vi "Marvin.vi"() -> ()   [LabVIEW 2017]
uses:
  PCAN_Driver/ControlCAN.llb/CAN Channel.ctl
  PCAN_Driver/ControlCAN.llb/DevType.ctl
  PCAN_Driver/ControlCAN.llb/VCI_INIT_CONFIG.ctl
  PCAN_Driver/ControlCAN.llb/InitFlag.ctl
  PCAN_Driver/ControlCAN.llb/Fliter.ctl
  PCAN_Driver/ControlCAN.llb/Mode.ctl
  <vilib>/Utility/miscctls.llb/LVMinMaxIncTypeDef.ctl
  PCAN_Driver/ControlCAN.llb/VCI_CAN_OBJ.ctl
  PCAN_Driver/ControlCAN.lvlib
panel:
  out "Array":u64[][](array[numeric]) format="%016x"
  out "Waveform Chart":dbl[](graph)
  out "Ambient Over temp":bool
  out "Ambient Sensor temp":bool
  out "Ambient Temperature":dbl
  in  "Motor Over Temp":bool
  in  "Speed control":bool
  out "Unit Adress":string
  in  "Serial Send":bool
  in  "Index":u16(ring) items=["1"=1, "2"=2, "3"=3]
  out "read buffer":string
  in  "SetGet":enum16{"Get", "Set"}(ring)
  in  "Function":T1(ring)
  in  "Value":dbl
  in  "Value 1/2":enum16{"1", "2"}(ring)
  out "Msg Count":u32
  in  "Param to Set":u16(ring) items=["EBAY 5F"=95, "AHU 3F"=63, "AHU 2F"=47]
  out "Unit Adress":u8
  out "Horizontal Progress Bar":i32(slide) min=0 max=48 scale=0.0..50.0
  out "character string":string
  in  "Set Param.":bool
  in  "Serial Monitor":bool caption="Graph Button"
  in  "Serial Com":bool
  in  "VISA resource name":refnum<visa-resource-name>="COM6"
  out "Serial Status":bool
  in  "Graph Button":bool
  in  "Refresh Button":bool
  out "Data Send":u64 format="%016x"
  in  "Motor Speed RPM":u16
  out "Under voltage/Over voltage":bool
  out "Speed error":bool
  out "Derated drive temp":bool
  out "Motor Over temperature":bool
  out "Commutation err":bool
  out "Motor Sensor temp Fauilre":bool
  out "Drive Over temperature":bool
  out "Drive Sensor temp Failure":bool
  out "Motor Phase Current RMS":dbl
  out "ECS State":u16
  out "Motor Speed RPM":dbl
  out "Motor Stator Temp.":dbl
  out "Power transistor Heat sink Temp.":dbl
  out "DC Current":dbl
  out "DC Voltage":dbl
  in  "Can Send":bool
  in  "Stop":bool
  out "Config_CANAT":T8 {"DevType" items=["USB-CAN"=3, "USB-CAN2"=4]; "CanIndex" items=["通道1", "通道2"]; "VCI_INIT_CONFIG"."Fliter" items=["接收所有类型"=3, "只接收标准帧"=4, "只接收扩展帧"=7]; "VCI_INIT_CONFIG"."Mode" items=["正常工作", "自测模式（环回）", "仅侦听模式"]; "VCI_INIT_CONFIG"."InitFlag" items=["使用Flash参数", "使用界面设置参数"]}
  in  "Channel 2":T3 caption="Channel" items=["Channel 1", "Channel 2"]
  out "CAN Status":bool
  # "ver 1.0"
  # "Marvin"
  # "REDLER TECHNOLOGIES LTD"
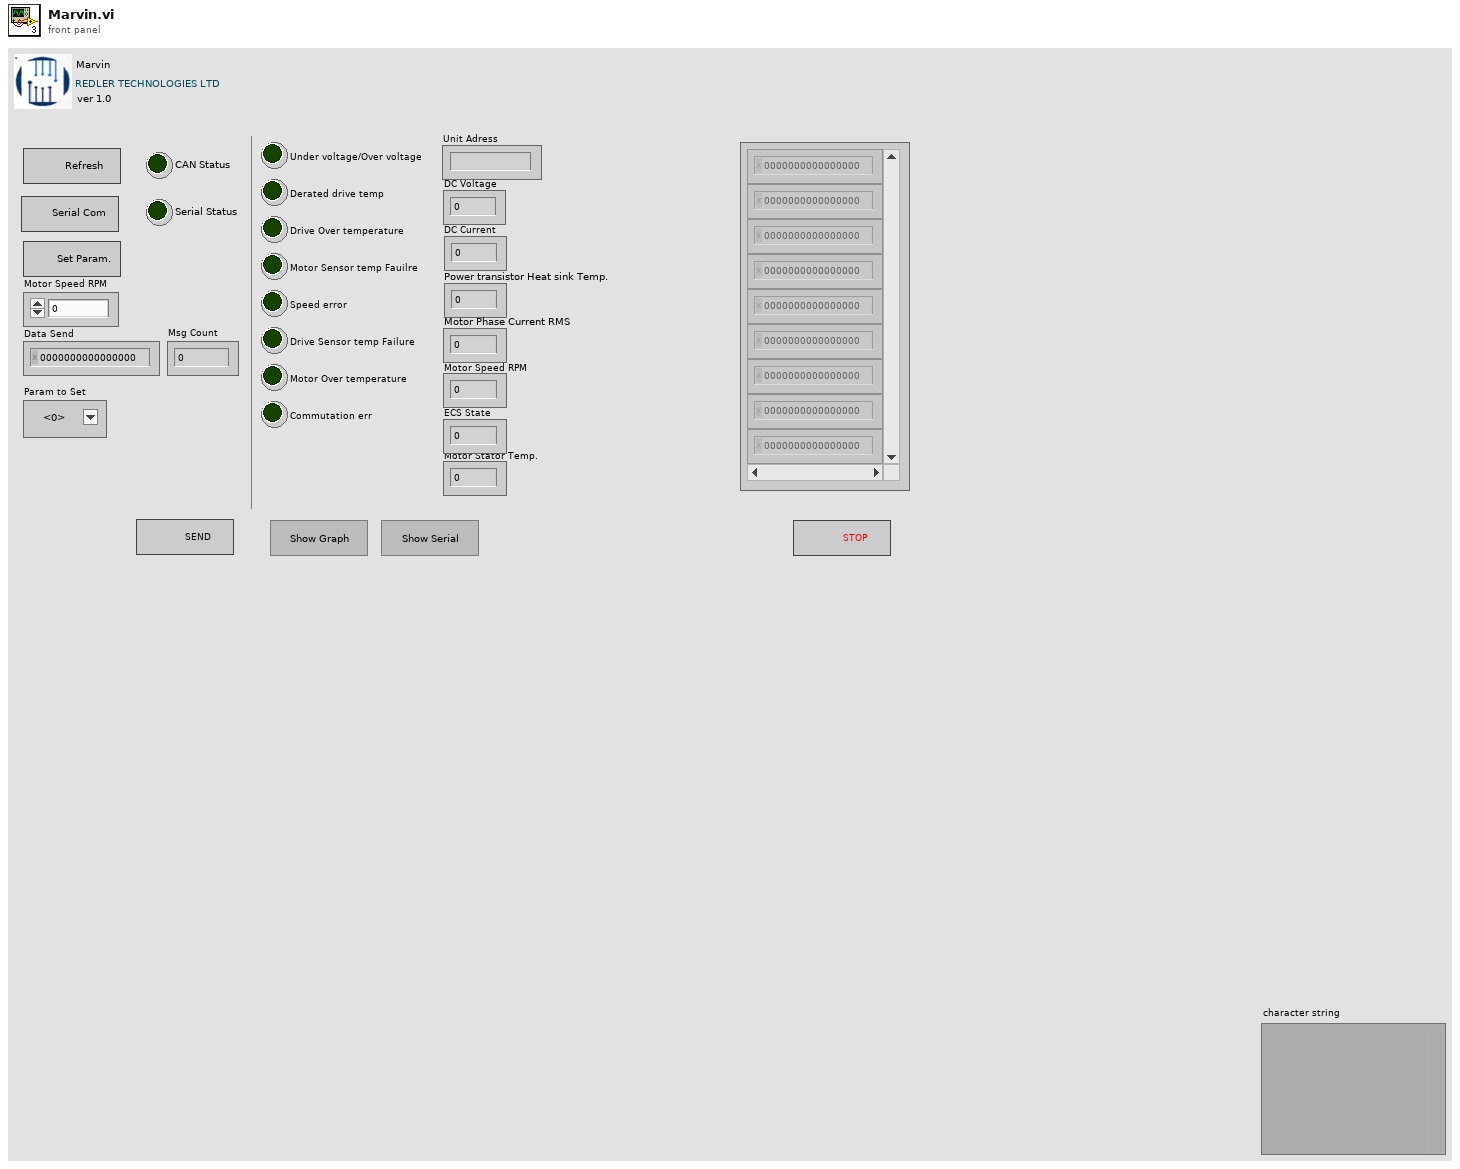
[diagram p1: front panel]
types:
  T1 = enum16{"Serial Number", "Temperature", "Unit Adress", "Calibration", "Velocity", "Version"}
  T2 = typedef "ControlCAN.lvlib/DevType.ctl" = u32
  T3 = typedef "ControlCAN.lvlib/CAN Channel.ctl" = u32
  T4 = typedef "ControlCAN.lvlib/VCI_INIT_CONFIG.ctl" = cluster{"AccCode":u32, "AccMask":u32, "InitFlag":T5, "Fliter":T6, "Timing0":u8, "Timing1":u8, "Mode":T7}
  T5 = typedef "ControlCAN.lvlib/InitFlag.ctl" = u32
  T6 = typedef "ControlCAN.lvlib/Fliter.ctl" = u8
  T7 = typedef "ControlCAN.lvlib/Mode.ctl" = u8
  T8 = cluster{"DevType":T2, "DevIndex":u32, "CanIndex":T3, "VCI_INIT_CONFIG":T4}
  T9 = cluster{"ID":u32, "MSGTYPE":u8, "LEN":u8, "aDATA":u8[]}[]
  T10 = cluster{"ID":u32, "MSGTYPE":u8, "LEN":u8, "aDATA":u8[]}
  T11 = enum8{"Enabled", "Disabled", "Disabled and Grayed Out"}
  T12 = typedef "LVMinMaxIncTypeDef.ctl" = cluster{"Minimum":dbl, "Maximum":dbl, "Increment":dbl}
  T13 = typedef "ControlCAN.lvlib/VCI_CAN_OBJ.ctl" = cluster{"ID":u32, "TimeStamp":u32, "TimeFlag":u8, "SendType":u8, "RemoteFlag":u8, "ExternFlag":u8, "DataLen":u8, "Data":u8[], "Reserved":u8[]}
  T14 = cluster{"Type":enum16{"接收", "发送"}, "Channel":T3, "Time":timestamp, "VCI_CAN_OBJ":T13}[]
  T15 = cluster{"Type":enum16{"接收", "发送"}, "Channel":T3, "Time":timestamp, "VCI_CAN_OBJ":T13}
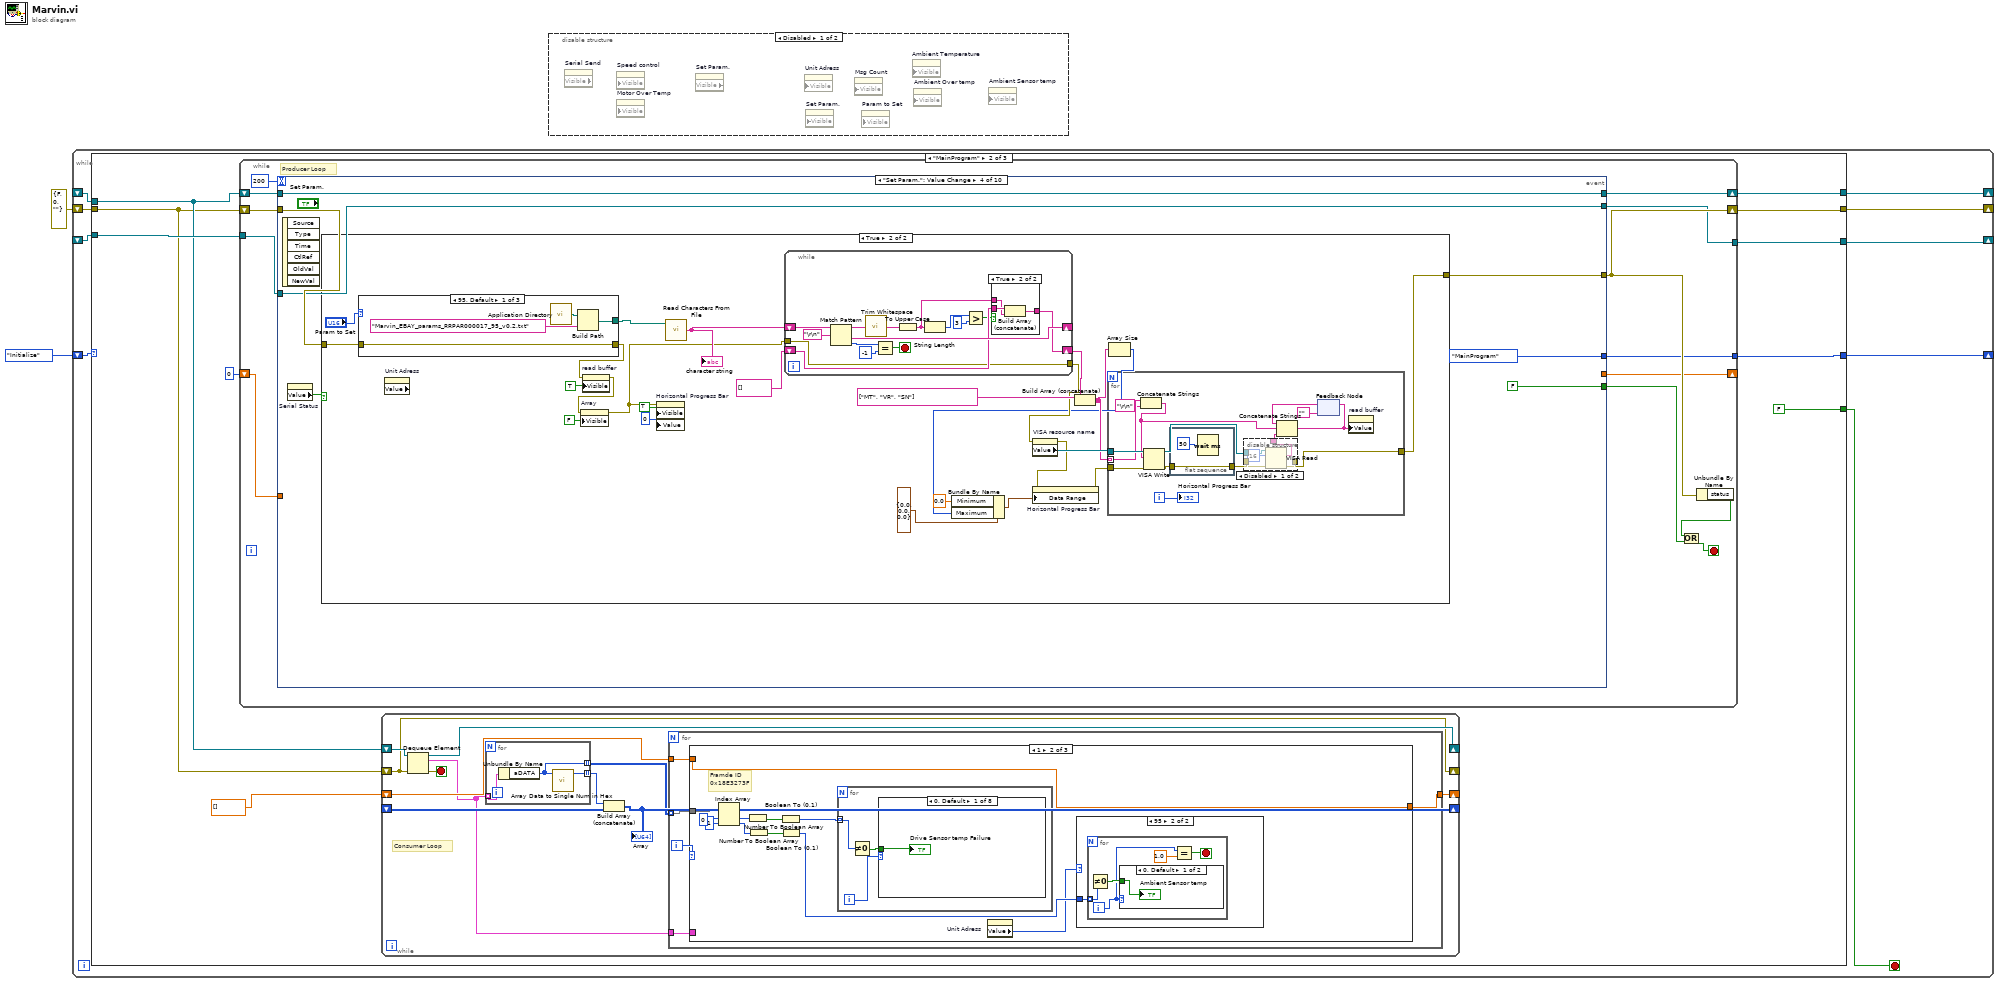
[diagram p0: block diagram]
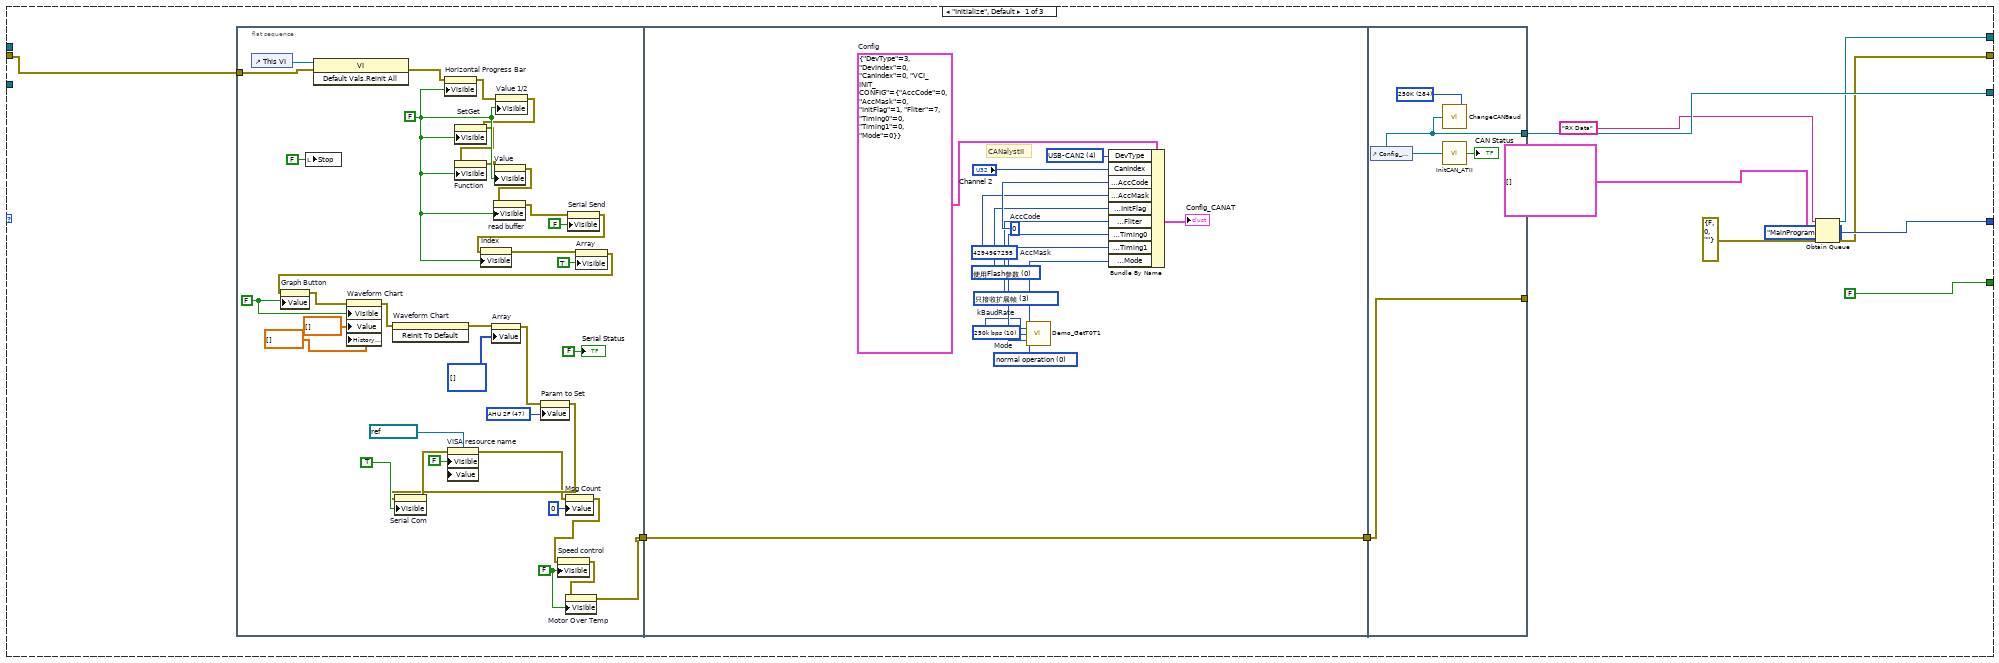
[diagram p3: hidden frame]
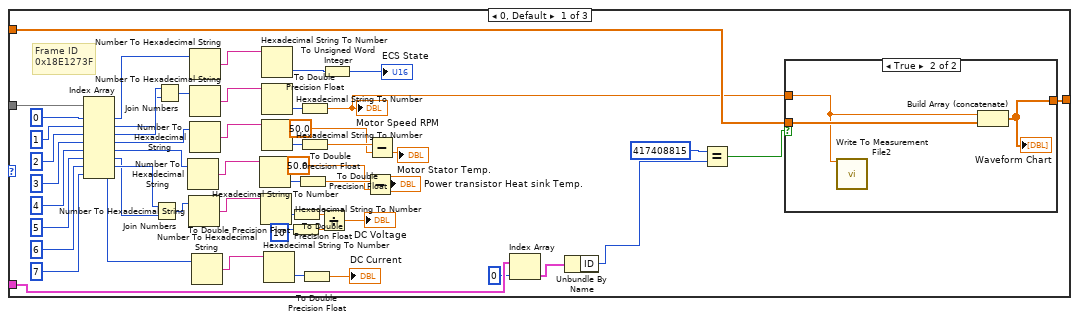
[diagram p4: hidden frame]
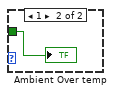
[diagram p7: hidden frame]
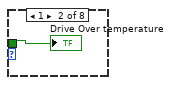
[diagram p8: hidden frame]
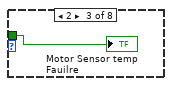
[diagram p9: hidden frame]
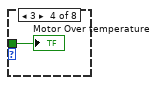
[diagram p10: hidden frame]
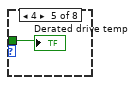
[diagram p11: hidden frame]
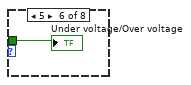
[diagram p12: hidden frame]
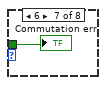
[diagram p13: hidden frame]
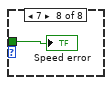
[diagram p14: hidden frame]
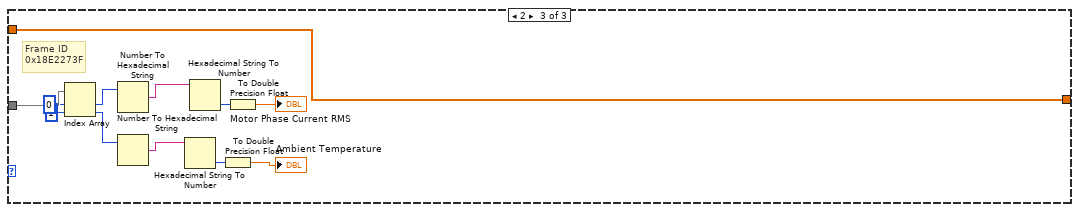
[diagram p15: hidden frame]
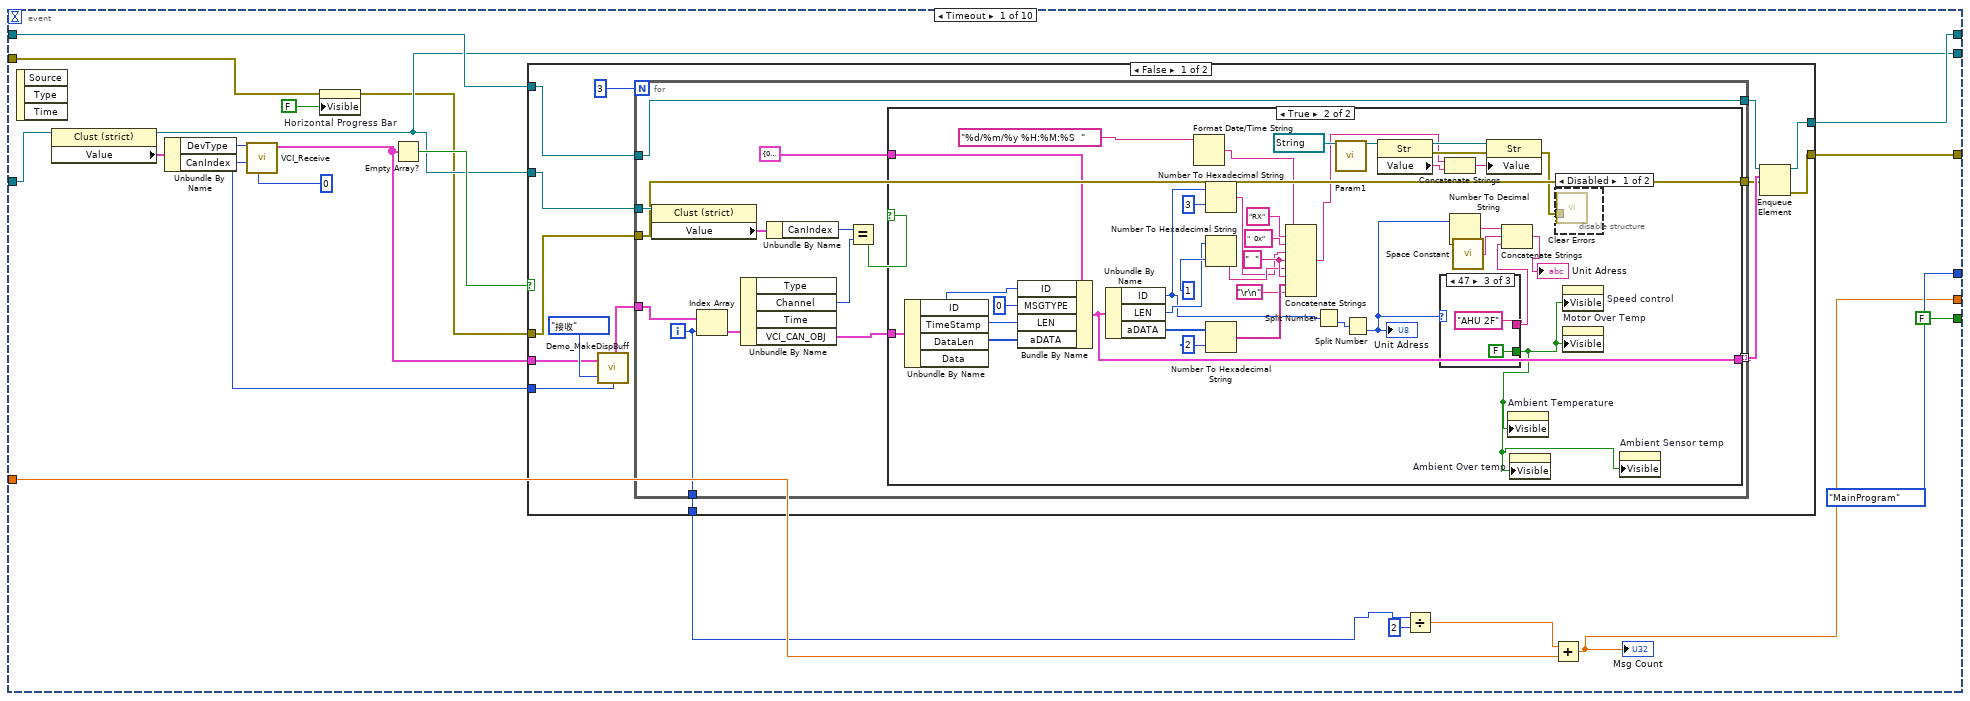
[diagram p16: hidden frame]
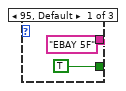
[diagram p18: hidden frame]
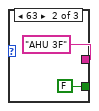
[diagram p19: hidden frame]
diagram:
  n1 = while {
    shift-right: [w6] -> _
    shift-left: enum16{"Stop", "MainProgram", "Initialize"}."Initialize" -> [w11]
    shift-right: [w10] -> _
    shift-left: _ -> [w9]
    shift-right: [w8] -> _
    shift-left: _ -> [w5]
    shift-right: [w7] -> _
    shift-left: errorcluster {"status"=FALSE, "code"=0, "source"=""} ("error out") -> [w4]
    stop <- w3 stop-if-true
    n2 = case shown="\"MainProgram\"" w11 {
      tunnel: [w22 w83 w734] -> w10
      tunnel: w9 -> [_ w86 w734]
      tunnel: [w18 w85 w735] -> w8
      tunnel: [w17 w84 w736] -> w7
      tunnel: [enum16{"Stop", "MainProgram", "Initialize"}."MainProgram" w82 enum16{"Stop", "MainProgram", "Initialize"}."Stop"] -> w6
      tunnel: w5 -> [_ w81 w735]
      tunnel: w4 -> [w15 w80 w737]
      tunnel: [FALSE ("Stop") FALSE ("Stop") w733] -> w3
      frame "Initialize", Default {
        n3 = flat-sequence {
          tunnel: w15 -> [w28]
          tunnel: [w24] -> w13
          tunnel: [w60] -> w14
          tunnel: w13 -> [w60]
          tunnel: [w74] -> w22
          tunnel: w14 -> [w73]
          tunnel: [w73] -> _
          frame #0 {
            w23 = FALSE ("Visible")
            w43 = u16 47 items=["EBAY 5F"=95, "AHU 3F"=63, "AHU 2F"=47] ("Param to Set")
            w46 = FALSE ("Visible")
            w50 = FALSE ("Graph Button")
            n4 = control-ref of="This VI"() -> (w59:refnum<vi>)
            n5 = local write "Stop"(FALSE ("Stop")) -> ()
            n6 = invoke class="VI" method="Default Vals.Reinit All"(reference=w59, error in=w28) -> (error out=w27:errorcluster)  [unwired: 1 in, 2 out]
            n7 = property on="Horizontal Progress Bar" class="Slide (strict)"(error in=w27, "Visible"=w46) -> (error out=w41:errorcluster)  [unwired: 1 in, 1 out]
            n8 = property on="Value 1/2" class="Enum (strict)"(error in=w41, "Visible"=w46) -> (error out=w40:errorcluster)  [unwired: 1 in, 1 out]
            n9 = property on="SetGet" class="Enum (strict)"(error in=w40, "Visible"=w46) -> (error out=w39:errorcluster)  [unwired: 1 in, 1 out]
            n10 = property on="Function" class="Enum (strict)"(error in=w39, "Visible"=w46) -> (error out=w38:errorcluster)  [unwired: 1 in, 1 out]
            n11 = property on="Value" class="DigNum (strict)"(error in=w38, "Visible"=w46) -> (error out=w37:errorcluster)  [unwired: 1 in, 1 out]
            n12 = property on="read buffer" class="Str"(error in=w37, "Visible"=w46) -> (error out=w36:errorcluster)  [unwired: 1 in, 1 out]
            n13 = property on="Serial Send" class="Bool"(error in=w36, "Visible"=FALSE) -> (error out=w35:errorcluster)  [unwired: 1 in, 1 out]
            n14 = property on="Index" class="Ring (strict)"(error in=w35, "Visible"=w46) -> (error out=w34:errorcluster)  [unwired: 1 in, 1 out]
            n15 = property on="Array" class="Arr (strict)"(error in=w34, "Visible"=TRUE) -> (error out=w33:errorcluster)  [unwired: 1 in, 1 out]
            n16 = property on="Graph Button" class="Bool (strict)"(error in=w33, "Value"=w50) -> (error out=w32:errorcluster)  [unwired: 1 in, 1 out]
            n17 = property on="Waveform Chart" class="WFChart (strict)"(error in=w32, "Visible"=w50, "Value"=dbl[] [] ("Waveform Chart"), "History Data"=dbl[] []) -> (error out=w53:errorcluster)  [unwired: 1 in, 1 out]
            n18 = invoke on="Waveform Chart" class="WFChart (strict)" method="Reinit To Default"(error in=w53) -> (error out=w54:errorcluster)  [unwired: 2 in, 2 out]
            n19 = property on="Array" class="Arr (strict)"(error in=w54, "Value"=u64[][] [] ("Array")) -> (error out=w31:errorcluster)  [unwired: 1 in, 1 out]
            n20 = property on="Param to Set" class="Ring (strict)"(error in=w31, "Value"=w43) -> (error out=w30:errorcluster)  [unwired: 1 in, 1 out]
            n21 = property on="Serial Com" class="Bool"(error in=w30, "Visible"=TRUE) -> (error out=w56:errorcluster)  [unwired: 1 in, 1 out]
            n22 = property on="VISA resource name" class="VISAName"(error in=w56, "Visible"=FALSE, "Value"=refnum<visa-resource-name> "COM1" ("VISA resource name")) -> (error out=w29:errorcluster)  [unwired: 1 in, 1 out]
            n23 = property on="Msg Count" class="DigNum (strict)"(error in=w29, "Value"=u32 0 ("Msg Count")) -> (error out=w26:errorcluster)  [unwired: 1 in, 1 out]
            n24 = property on="Speed control" class="Bool (strict)"(error in=w26, "Visible"=w23) -> (error out=w25:errorcluster)  [unwired: 1 in, 1 out]
            n25 = property on="Motor Over Temp" class="Bool (strict)"(error in=w25, "Visible"=w23) -> (error out=w24:errorcluster)  [unwired: 1 in, 1 out]
            "Serial Status" <- FALSE ("Serial Status")
          }
          frame #1 {
            w64 = u32 4294967295  # AccMask
            w63 = T5 0 items=["使用Flash参数", "使用界面设置参数"] ("InitFlag")
            w61 = T7 0 items=["normal operation", "Listen-only mode", "test mode"]  # Mode
            w62 = T6 3 items=["接收所有类型"=1, "只接收标准帧"=2, "只接收扩展帧"=3] ("Fliter")
            w68 = u8 10 items=["5k bps"=1, "10k bps"=2, "20k bps"=3, "40k bps"=4, "50k bps"=5, "80k bps"=6, "100k bps"=7, "125k bps"=8, "200k bps"=9, "250k bps"=10, "400k bps"=11, "500k bps"=12, "666k bps"=13, "800k bps"=14, "1000k bps"=15, "33.33k bps"=16, "66.66k bps"=17, "83.33k bps"=18]  # kBaudRate
            w65 = u32 0  # AccCode
            w66 = T2 4 items=["USB-CAN"=3, "USB-CAN2"=4] ("DevType")
            w67 = T8 {"DevType"=3, "DevIndex"=0, "CanIndex"=0, "VCI_INIT_CONFIG"={"AccCode"=0, "AccMask"=0, "InitFlag"=1, "Fliter"=7, "Timing0"=0, "Timing1"=0, "Mode"=0}}  # Config
            # "CANalystII"
            n26 = call "Demo_GetT0T1.vi"("kBaudRate"=w68) -> ("Timing0"=w70:u8, "Timing1"=w71:u8)
            n27 = Bundle By Name(cluster=w67, "DevType"=w66, "CanIndex"="Channel 2", "VCI_INIT_CONFIG.AccCode"=w65, "VCI_INIT_CONFIG.AccMask"=w64, "VCI_INIT_CONFIG.InitFlag"=w63, "VCI_INIT_CONFIG.Fliter"=w62, "VCI_INIT_CONFIG.Timing0"=w70, "VCI_INIT_CONFIG.Timing1"=w71, "VCI_INIT_CONFIG.Mode"=w61) -> (→"Config_CANAT":T8)
          }
          frame #2 {
            w75 = u16 284 items=["1M"=20, "500K"=28, "250K"=284, "125K"=796, "100K"=17199, "50K"=18223, "20K"=21295, "10K"=26415, "5K"=32639] ("baud in")
            n28 = control-ref of="Config_CANAT"() -> (w74:refnum<vi>)
            n29 = call "ChangeCANBaud.vi"("baud in"=w75, "reference"=w74) -> ()
            n30 = call "InitCAN_ATII.vi"("Config"=w74) -> ("Sts"=→"CAN Status":bool)
          }
        }
        n31 = Obtain Queue(name (unnamed)="RX Data", element data type=T9 [], error in (no error)=errorcluster {"status"=FALSE, "code"=0, "source"=""}) -> (queue out=w18:refnum<queue>, error out=w17:errorcluster)  [unwired: 2 in, 1 out]
      }
      frame "MainProgram" {
        n32 = while {
          shift-right: [w210] -> w84
          shift-left: w80 -> [w212]
          shift-right: [w211] -> w85
          shift-left: w81 -> [w213]
          tunnel: w86 -> [w214]
          tunnel: [w207] -> w83
          tunnel: [w206] -> w82
          shift-right: [w204] -> _
          shift-left: 0 -> [w205]
          stop <- w215 stop-if-true
          # "Producer Loop"
          n33 = event shown="[3] \"Set Param.\": Value Change" {
            selector: _ -> [_ _ _ _ _ _ _ _ _ _]
            dyn-events: _ -> [_ _ _ _ _ _ _ _ _ _]
            timeout: 200 -> [_ _ _ _ _ _ _ _ _ _]
            tunnel: w214 -> [w234 w315 w356 w542 w636 w686 w698 w711 w725 w730]
            tunnel: w213 -> [w231 w319 w357 w541 w657 w687 w697 w712 w722 w727]
            tunnel: w212 -> [w223 w316 w358 w543 w656 w688 w693 w704 w721 w728]
            tunnel: [w229 w319 w357 w541 w657 w687 w697 w712 w720 w727] -> w211
            tunnel: [w228 w314 w355 w538 w656 w688 w690 w701 w718 w726] -> w210
            tunnel: [FALSE ("Stop") FALSE ("Stop") FALSE ("Stop") FALSE ("Stop") FALSE ("Stop") FALSE ("Stop") FALSE ("Stop") FALSE ("Stop") TRUE ("Stop") TRUE ("Stop")] -> w208
            tunnel: [w227 w315 w356 w542 w636 w686 w698 w711 w725 w730] -> w207
            tunnel: [enum16{"Stop", "MainProgram", "Initialize"}."MainProgram" enum16{"Stop", "MainProgram", "Initialize"}."MainProgram" enum16{"Stop", "MainProgram", "Initialize"}."MainProgram" enum16{"Stop", "MainProgram", "Initialize"}."MainProgram" enum16{"Stop", "MainProgram", "Initialize"}."MainProgram" enum16{"Stop", "MainProgram", "Initialize"}."MainProgram" enum16{"Stop", "MainProgram", "Initialize"}."MainProgram" enum16{"Stop", "MainProgram", "Initialize"}."MainProgram" enum16{"Stop", "MainProgram", "Initialize"}."Stop" enum16{"Stop", "MainProgram", "Initialize"}."Initialize"] -> w206
            tunnel: w205 -> [w222 _ _ _ _ _ _ _ _ _]
            tunnel: [w221 _ _ _ _ _ _ _ _ _] -> w204
            event Timeout {
              n34 = event-data() -> ()  [unwired: 1 in, 3 out]
              n35 = property class="Clust (strict)"(reference=w234) -> (reference out=w227:refnum<vi>, "Value"=w235:T8)  [unwired: 1 in, 1 out]
              n36 = Unbundle By Name(w235) -> ("DevType"=w236:T2, "CanIndex"=w232:T3)
              n37 = call "VCI_Receive.vi"("CANIndex"=w232, "DevIndex"=u32 0, "DevType"=w236) -> ("Recieve"=w230:T13[])  [unwired: 3 in, 5 out]
              n38 = property on="Horizontal Progress Bar" class="Slide (strict)"(error in=w223, "Visible"=FALSE) -> (error out=w217:errorcluster)  [unwired: 1 in, 1 out]
              n39 = Empty Array?(array=w230) -> (empty?=w233:bool)
              n40 = case shown="False" w233 {
                tunnel: w232 -> [w249 _]
                tunnel: w227 -> [w247 _]
                tunnel: w231 -> [w246 w312]
                tunnel: w217 -> [w245 w311]
                tunnel: w230 -> [w250 _]
                tunnel: [w240 w311] -> w228
                tunnel: [w239 w312] -> w229
                tunnel: [w238 0] -> w218
                frame False {
                  n41 = call "Demo_MakeDispBuff.vi"("Channel"=w249, "Type"=enum16{"接收", "发送"}."接收", "OBJs"=w250) -> ("Buffer"=w248:T14)
                  n42 = for {
                    N: 3 -> [_]
                    tunnel: w248 -> [w264]
                    tunnel: w247 -> [w263]
                    tunnel: w246 -> [w254]
                    tunnel: w245 -> [w253]
                    tunnel: [w256] -> w243 mode=indexing
                    tunnel: [w254] -> w242
                    tunnel: [w253] -> w241
                    tunnel: [w252] -> w238
                    i -> [w252]
                    n43 = property class="Clust (strict)"(reference=w263) -> ("Value"=w261:T8)  [unwired: 1 in, 2 out]
                    n44 = Index Array(array=w264, index=w252) -> (element=w257:T15)
                    n45 = Unbundle By Name(w257) -> ("Channel"=w259:T3, "VCI_CAN_OBJ"=w262:T13)  [unwired: 2 out]
                    n46 = Unbundle By Name(w261) -> ("CanIndex"=w260:T3)
                    n47 = Equal?(x=w260, y=w259) -> (x = y?=w258:bool)
                    n48 = case shown="True" w258 {
                      tunnel: w262 -> [_ w302]
                      tunnel: [w265 w278] -> w256
                      tunnel: T10 {"ID"=0, "MSGTYPE"=0, "LEN"=0, "aDATA"=[]} ("Msg") -> [w265 w277]
                      frame False {
                      }
                      frame True {
                        w289 = "  " ("string")
                        n49 = Unbundle By Name(w302) -> ("ID"=w274:u32, "DataLen"=w301:u8, "Data"=w279:u8[])  [unwired: 1 out]
                        n50 = Bundle By Name(cluster=w277, "ID"=w274, "MSGTYPE"=u8 0, "LEN"=w301, "aDATA"=w279) -> (w278:T10)
                        n51 = Unbundle By Name(w278) -> ("ID"=w272:u32, "LEN"=w284:u8, "aDATA"=w290:u8[])
                        n52 = Format Date/Time String(time format string (%c)="%d/%m/%y %H:%M:%S  ") -> (date/time string=w299:string)  [unwired: 2 in]
                        n53 = Number To Hexadecimal String(1:i16 3 ("width (-)"), 2:w272) -> (0:w276:string)
                        n54 = Number To Hexadecimal String(1:i16 1 ("width (-)"), 2:w284) -> (0:w288:string)
                        n55 = Number To Hexadecimal String(1:i16 2 ("width (-)"), 2:w290) -> (0:w291:string[])
                        n56 = Concatenate Strings(w299, "RX" ("string"), "  0x" ("string"), w276, w289, w288, w289, w291, "\r\n") -> (w275:string)
                        n57 = Split Number(x=w272) -> (lo(x)=w273:u16)  [unwired: 1 out]
                        n58 = call "Param1.vi"("str"=refnum<vi> refnum) -> ("str out"=w293:refnum<vi>)  [unwired: 17 in, 1 out]
                        n59 = Split Number(x=w273) -> (lo(x)=w271:u8)  [unwired: 1 out]
                        "Unit Adress" <- w271
                        n60 = property class="Str"(reference=w293) -> (reference out=w295:refnum<vi>, error out=w281:errorcluster, "Value"=w296:string)  [unwired: 1 in]
                        n61 = case shown="47" w271 {
                          tunnel: ["EBAY 5F" "AHU 3F" "AHU 2F"] -> w269
                          tunnel: [TRUE FALSE FALSE] -> w266
                          frame 95, Default {
                          }
                          frame 63 {
                          }
                          frame 47 {
                          }
                        }
                        n62 = Concatenate Strings(w275, w296) -> (w294:string)
                        n63 = Number To Decimal String(number=w271) -> (decimal integer string=w270:string)  [unwired: 1 in]
                        n64 = call <vilib>:"Space Constant.vi"() -> ("String"=w267:string)
                        n65 = property class="Str"(reference=w295, error in=w281, "Value"=w294) -> (error out=w280:errorcluster)  [unwired: 1 out]
                        n66 = Concatenate Strings(w270, w267, w269) -> (→"Unit Adress":string)
                        n67 = property on="Ambient Temperature" class="DigNum (strict)"("Visible"=w266) -> ()  [unwired: 2 in, 2 out]
                        n68 = property on="Ambient Over temp" class="Bool (strict)"("Visible"=w266) -> ()  [unwired: 2 in, 2 out]
                        n69 = disable-structure shown="Disabled" {
                          disable-tunnel: w280 -> [w309 _]
                          frame Disabled {
                            n70 = call <vilib>:"Clear Errors.vi"("error in (no error)"=w309) -> ()  [unwired: 5 in, 2 out]
                          }
                          frame Enabled {
                          }
                        }
                        n71 = property on="Speed control" class="Bool (strict)"("Visible"=w266) -> ()  [unwired: 2 in, 2 out]
                        n72 = property on="Motor Over Temp" class="Bool (strict)"("Visible"=w266) -> ()  [unwired: 2 in, 2 out]
                        n73 = property on="Ambient Sensor temp" class="Bool (strict)"("Visible"=w266) -> ()  [unwired: 2 in, 2 out]
                      }
                    }
                  }
                  n74 = Enqueue Element(queue=w242, element=w243, error in (no error)=w241) -> (queue out=w239:refnum<queue>, error out=w240:errorcluster)  [unwired: 2 out]
                }
                frame True {
                }
              }
              n75 = Divide(x=w218, y=u32 2) -> (x/y=w219:dbl)
              n76 = Add(x=w219, y=w222) -> (x+y=w221:dbl)
              "Msg Count" <- w221
            }
            event "Serial Monitor": Value Change {
              n77 = event-data() -> ()  [unwired: 1 in, 6 out]
              n78 = property on="Serial Status" class="Bool (strict)"() -> ("Value"=w313:bool)  [unwired: 2 in, 2 out]
              n79 = case shown="True" w313 {
                tunnel: w316 -> [w321 w332]
                tunnel: [w320 w338] -> w314
                frame False {
                  n80 = call "Display Message to User3"("error in (no error)"=w321) -> ("error out"=w320:errorcluster)  [unwired: 9 in, 1 out]
                }
                frame True {
                  w334 = FALSE ("Visible")
                  w335 = u16 1 items=["1"=1, "2"=2, "3"=3] ("Index")
                  n81 = property on="Index" class="Ring (strict)"(error in=w332, "Value"=w335) -> (error out=w331:errorcluster)  [unwired: 1 in, 1 out]
                  n82 = property on="Value 1/2" class="Enum (strict)"(error in=w331, "Visible"=w334) -> (error out=w330:errorcluster)  [unwired: 1 in, 1 out]
                  n83 = property on="Value" class="DigNum (strict)"(error in=w330, "Visible"=w334) -> (error out=w329:errorcluster)  [unwired: 1 in, 1 out]
                  n84 = property on="SetGet" class="Enum (strict)"(error in=w329, "Value"=enum16{"Get", "Set"}."Get" ("SetGet")) -> (error out=w327:errorcluster)  [unwired: 1 in, 1 out]
                  n85 = property on="Serial Send" class="Bool"(error in=w327, "Visible"=FALSE) -> (error out=w326:errorcluster)  [unwired: 1 in, 1 out]
                  n86 = property on="Function" class="Enum (strict)"(error in=w326, "Value"=T1."Serial Number" ("Function")) -> (error out=w324:errorcluster)  [unwired: 1 in, 1 out]
                  n87 = property on="Index" class="Ring (strict)"(error in=w324, "DisabledEnum"=T11."Disabled and Grayed Out" ("Disabled")) -> (error out=w322:errorcluster)  [unwired: 1 in, 1 out]
                  n88 = case shown="False" "Serial Monitor" {
                    selector: "Serial Monitor" -> [w339 w345]
                    tunnel: w322 -> [w343 w350]
                    tunnel: [w342 w348] -> w338
                    tunnel: [FALSE TRUE] -> w336
                    frame False {
                      (unwired) FALSE ("Visible")
                      n89 = Not(x=w339) -> (.not. x?=w340:bool)
                      n90 = property on="Array" class="Arr (strict)"(error in=w343, "Visible"=w340) -> (error out=w344:errorcluster)  [unwired: 1 in, 1 out]
                      n91 = property on="Serial Monitor" class="Bool (strict)"(error in=w344, "Value"=w339) -> (error out=w342:errorcluster)  [unwired: 1 in, 1 out]
                    }
                    frame True {
                      (unwired) FALSE ("Visible")
                      n92 = Not(x=w345) -> (.not. x?=w346:bool)
                      n93 = property on="Array" class="Arr (strict)"(error in=w350, "Visible"=w346) -> (error out=w349:errorcluster)  [unwired: 1 in, 1 out]
                      n94 = property on="Serial Monitor" class="Bool (strict)"(error in=w349, "Value"=w345) -> (error out=w348:errorcluster)  [unwired: 1 in, 1 out]
                    }
                  }
                  n95 = property on="SetGet" class="Enum (strict)"("Visible"=w336) -> ()  [unwired: 2 in, 2 out]
                  n96 = property on="Function" class="Enum (strict)"("Visible"=w336) -> ()  [unwired: 2 in, 2 out]
                  n97 = property on="Serial Send" class="Bool"("Visible"=w336) -> ()  [unwired: 2 in, 2 out]
                  n98 = property on="read buffer" class="Str"("Visible"=w336) -> ()  [unwired: 2 in, 2 out]
                  n99 = property on="Index" class="Ring (strict)"("Visible"=w336) -> ()  [unwired: 2 in, 2 out]
                }
              }
            }
            event "Serial Send": Value Change {
              n100 = event-data() -> ()  [unwired: 1 in, 6 out]
              n101 = property on="VISA resource name" class="VISAName"() -> ("Value"=w359:refnum<visa-resource-name>)  [unwired: 2 in, 2 out]
              n102 = case shown="\"Set\"" "SetGet" {
                tunnel: "Function" -> [w365 w444]
                tunnel: w359 -> [w373 w459]
                tunnel: w358 -> [w369 w443]
                tunnel: "Value" -> [_ w458]
                tunnel: "Value 1/2" -> [_ w456]
                tunnel: "Index" -> [w366 w453]
                tunnel: [w372 w451] -> _
                tunnel: [w371 w450] -> w355
                tunnel: [w367 w448] -> w354
                frame "Get", Default {
                  w370 = FALSE ("Visible")
                  n103 = property on="Value" class="DigNum (strict)"(error in=w369, "Visible"=w370) -> (error out=w368:errorcluster)  [unwired: 1 in, 1 out]
                  n104 = property on="Value 1/2" class="Enum (strict)"(error in=w368, "Visible"=w370) -> (error out=w364:errorcluster)  [unwired: 1 in, 1 out]
                  n105 = case shown="\"Version\"" w365 {
                    tunnel: w373 -> [w377 w393 w407 w415 w421 w430]
                    tunnel: w364 -> [w375 w384 w397 w410 w419 w428]
                    tunnel: [w377 w393 w407 w415 w421 w430] -> w372
                    tunnel: [w380 w394 w408 w416 w425 w431] -> w371
                    tunnel: [w379 w395 w406 w417 w426 w432] -> w367
                    tunnel: w366 -> [_ w388 w399 _ _ _]
                    frame "Serial Number", Default {
                      n106 = property on="Index" class="Ring (strict)"(error in=w375, "DisabledEnum"=T11."Disabled and Grayed Out" ("Disabled")) -> (error out=w374:errorcluster)  [unwired: 1 in, 1 out]
                      n107 = Concatenate Strings("SN" ("string"), "\r\n" ("write buffer")) -> (w378:string)
                      n108 = call "Serial.vi"("error in (no error)"=w374, "write buffer"=w378, "VISA resource name"=w377) -> ("error out"=w380:errorcluster, "read buffer"=w379:string)  [unwired: 7 in]
                    }
                    frame "Temperature" {
                      n109 = Number To Decimal String(number=w388) -> (decimal integer string=w387:string)  [unwired: 1 in]
                      n110 = property on="Index" class="Ring (strict)"(error in=w384, "DisabledEnum"=T11."Enabled" ("Disabled")) -> (error out=w383:errorcluster)  [unwired: 1 in, 1 out]
                      n111 = Concatenate Strings("TA" ("string"), "[", w387, "]", "\r\n" ("write buffer")) -> (w389:string)
                      n112 = call "Serial.vi"("error in (no error)"=w383, "write buffer"=w389, "VISA resource name"=w393) -> ("error out"=w394:errorcluster, "read buffer"=w395:string)  [unwired: 7 in]
                    }
                    frame "Unit Adress" {
                      n113 = Number To Decimal String(number=w399) -> (decimal integer string=w405:string)  [unwired: 1 in]
                      n114 = property on="Index" class="Ring (strict)"(error in=w397, "DisabledEnum"=T11."Enabled" ("Disabled")) -> (error out=w396:errorcluster)  [unwired: 1 in, 1 out]
                      n115 = Concatenate Strings("UA" ("string"), "[", w405, "]", "\r\n" ("write buffer")) -> (w400:string)
                      n116 = call "Serial.vi"("error in (no error)"=w396, "write buffer"=w400, "VISA resource name"=w407) -> ("error out"=w408:errorcluster, "read buffer"=w406:string)  [unwired: 7 in]
                    }
                    frame "Calibration" {
                      n117 = property on="Index" class="Ring (strict)"(error in=w410, "DisabledEnum"=T11."Disabled and Grayed Out" ("Disabled")) -> (error out=w409:errorcluster)  [unwired: 1 in, 1 out]
                      n118 = Concatenate Strings("CC" ("string"), "\r\n" ("write buffer")) -> (w413:string)
                      n119 = call "Serial.vi"("error in (no error)"=w409, "write buffer"=w413, "VISA resource name"=w415) -> ("error out"=w416:errorcluster, "read buffer"=w417:string)  [unwired: 7 in]
                    }
                    frame "Velocity" {
                      n120 = property on="Index" class="Ring (strict)"(error in=w419, "DisabledEnum"=T11."Disabled and Grayed Out" ("Disabled")) -> (error out=w418:errorcluster)  [unwired: 1 in, 1 out]
                      n121 = Concatenate Strings("VC" ("string"), "\r\n" ("write buffer")) -> (w422:string)
                      n122 = call "Serial.vi"("error in (no error)"=w418, "write buffer"=w422, "VISA resource name"=w421) -> ("error out"=w425:errorcluster, "read buffer"=w426:string)  [unwired: 7 in]
                    }
                    frame "Version" {
                      n123 = property on="Index" class="Ring (strict)"(error in=w428, "DisabledEnum"=T11."Disabled and Grayed Out" ("Disabled")) -> (error out=w427:errorcluster)  [unwired: 1 in, 1 out]
                      n124 = Concatenate Strings("VR" ("string"), "\r\n" ("write buffer")) -> (w433:string)
                      n125 = call "Serial.vi"("error in (no error)"=w427, "write buffer"=w433, "VISA resource name"=w430) -> ("error out"=w431:errorcluster, "read buffer"=w432:string)  [unwired: 7 in]
                    }
                  }
                }
                frame "Set" {
                  w445 = "EP=1\r\n" ("write buffer")
                  n126 = To Unsigned Long Integer(number=w458) -> (unsigned 32bit integer=w454:u32)
                  n127 = Number To Decimal String(number=w453) -> (decimal integer string=w452:string)  [unwired: 1 in]
                  n128 = Number To Decimal String(number=w456) -> (decimal integer string=w455:string)  [unwired: 1 in]
                  n129 = case shown="\"Serial Number\", Default" w444 {
                    tunnel: w443 -> [w467 w471 w475 w479 w483 w487]
                    tunnel: [FALSE TRUE TRUE FALSE FALSE FALSE] -> w441
                    tunnel: [TRUE TRUE TRUE FALSE TRUE FALSE] -> w440
                    tunnel: [FALSE FALSE FALSE TRUE FALSE FALSE] -> w439
                    tunnel: [w467 w471 w475 w479 w483 w487] -> w436
                    frame "Serial Number", Default {
                    }
                    frame "Temperature" {
                    }
                    frame "Unit Adress" {
                    }
                    frame "Calibration" {
                    }
                    frame "Velocity" {
                    }
                    frame "Version" {
                    }
                  }
                  n130 = Number To Decimal String(number=w454) -> (decimal integer string=w457:string)  [unwired: 1 in]
                  n131 = flat-sequence {
                    tunnel: w463 -> [w490]
                    tunnel: [w490] -> w461
                    frame #0 {
                      n132 = Wait (ms)(milliseconds to wait=u32 50) -> ()  [unwired: 1 out]
                    }
                  }
                  n133 = property on="Index" class="Ring (strict)"(error in=w436, "Visible"=w441) -> (error out=w442:errorcluster)  [unwired: 1 in, 1 out]
                  n134 = property on="Value" class="DigNum (strict)"(error in=w442, "Visible"=w440) -> (error out=w438:errorcluster)  [unwired: 1 in, 1 out]
                  n135 = property on="Value 1/2" class="Enum (strict)"(error in=w438, "Visible"=w439) -> (error out=w437:errorcluster)  [unwired: 1 in, 1 out]
                  n136 = VISA Write(VISA resource name=w459, write buffer=w445, error in (no error)=w437) -> (error out=w463:errorcluster)  [unwired: 2 out]
                  n137 = case shown="\"Temperature\"" w444 {
                    tunnel: [w493 w499 w508 w516 w534] -> w446
                    tunnel: w461 -> [w492 w498 w507 w521 w525]
                    tunnel: [w492 w498 w507 w521 w522] -> w460
                    tunnel: w457 -> [w494 w500 w513 _ _]
                    tunnel: w455 -> [_ _ _ w517 _]
                    tunnel: w454 -> [_ _ _ _ w526]
                    tunnel: w452 -> [_ w501 w511 _ _]
                    frame "Serial Number", Default {
                      n138 = Concatenate Strings("SN" ("write buffer"), "=" ("string"), w494, "\r\n" ("write buffer")) -> (w493:string)
                    }
                    frame "Temperature" {
                      n139 = Concatenate Strings("TA" ("string"), "[", w501, "]", "=" ("string"), w500, "\r\n" ("write buffer")) -> (w499:string)
                    }
                    frame "Unit Adress" {
                      n140 = Concatenate Strings("UA" ("string"), "[", w511, "]", "=" ("string"), w513, "\r\n" ("write buffer")) -> (w508:string)
                    }
                    frame "Calibration" {
                      n141 = Concatenate Strings("CC" ("string"), "=" ("string"), w517, "\r\n" ("write buffer")) -> (w516:string)
                    }
                    frame "Velocity" {
                      n142 = In Range and Coerce(upper limit=u16 18001, x=w526, lower limit=u16 0) -> (coerced(x)=w532:u32, In Range?=w530:bool)
                      n143 = Not(x=w530) -> (.not. x?=w531:bool)
                      n144 = Select(t=w532, s=w530, f=u16 0) -> (s? t:f=w524:u32)
                      n145 = call "Display Message to User2"("error in (no error)"=w525, "Enable"=w531) -> ("error out"=w522:errorcluster)  [unwired: 8 in, 1 out]
                      n146 = Number To Decimal String(number=w524) -> (decimal integer string=w523:string)  [unwired: 1 in]
                      n147 = Concatenate Strings("VC" ("write buffer"), "=" ("string"), w523, "\r\n" ("write buffer")) -> (w534:string)
                    }
                  }
                  n148 = VISA Write(VISA resource name=w459, write buffer=w446, error in (no error)=w460) -> (VISA resource name out=w451:refnum<visa-resource-name>, error out=w462:errorcluster)  [unwired: 1 out]
                  n149 = flat-sequence {
                    tunnel: w462 -> [w488]
                    tunnel: [w488] -> w450
                    frame #0 {
                      n150 = Wait (ms)(milliseconds to wait=u32 50) -> ()  [unwired: 1 out]
                    }
                  }
                  n151 = feedback #1("") -> (w447:string)
                  n152 = Concatenate Strings(w447, w445, w446) -> (w448:string)
                  n153 = feedback-in #1(w448) -> ()
                }
              }
              "read buffer" <- w354
            }
            event "Set Param.": Value Change {
              n154 = event-data() -> ()  [unwired: 1 in, 6 out]
              n155 = property on="Serial Status" class="Bool (strict)"() -> ("Value"=w537:bool)  [unwired: 2 in, 2 out]
              n156 = case shown="True" w537 {
                tunnel: w543 -> [w545 w569]
                tunnel: [w544 w551] -> w538
                frame False {
                  n157 = call "Display Message to User4"("error in (no error)"=w545) -> ("error out"=w544:errorcluster)  [unwired: 9 in, 1 out]
                }
                frame True {
                  n158 = case shown="95, Default" "Param to Set" {
                    tunnel: [w611 w615 w619] -> w566
                    tunnel: w569 -> [w610 w614 w618]
                    tunnel: [w610 w614 w618] -> w552
                    frame 95, Default {
                      n159 = call <vilib>:"Application Directory.vi"() -> ("Application Directory"=w613:path)
                      n160 = Build Path(base path=w613, name or relative path="Marvin_EBAY_params_RRPAR000017_95_v0.2.txt") -> (appended path=w611:path)
                    }
                    frame 63 {
                      n161 = call <vilib>:"Application Directory.vi"() -> ("Application Directory"=w617:path)
                      n162 = Build Path(base path=w617, name or relative path="Marvin_AHU_params_RRPAR000016_63_v0.2.txt") -> (appended path=w615:path)
                    }
                    frame 47 {
                      n163 = call <vilib>:"Application Directory.vi"() -> ("Application Directory"=w621:path)
                      n164 = Build Path(base path=w621, name or relative path="Marvin_AHU_params_RRPAR000015_47_v0.2.txt") -> (appended path=w619:path)
                    }
                  }
                  n165 = property on="Unit Adress" class="DigNum (strict)" props=["Value"]() -> ()  [unwired: 2 in, 3 out]
                  n166 = property on="read buffer" class="Str"(error in=w552, "Visible"=TRUE) -> (error out=w547:errorcluster)  [unwired: 1 in, 1 out]
                  n167 = property on="Array" class="Arr (strict)"(error in=w547, "Visible"=FALSE) -> (error out=w546:errorcluster)  [unwired: 1 in, 1 out]
                  n168 = property on="Horizontal Progress Bar" class="Slide (strict)"(error in=w546, "Visible"=TRUE, "Value"=u8 0 ("Horizontal Progress Bar")) -> ()  [unwired: 1 in, 2 out]
                  n169 = call <vilib>:"Read Characters From File.vi"("file path (dialog if empty)"=w566) -> ("character string"=w567:string)  [unwired: 5 in, 3 out]
                  "character string" <- w567
                  n170 = while {
                    shift-right: [w602] -> _
                    shift-left: w567 -> [w603]
                    shift-right: [w598] -> w549
                    shift-left: string[] [] -> [w599]
                    tunnel: w546 -> [w591]
                    tunnel: [w591] -> w563
                    stop <- w604 stop-if-true
                    n171 = Match Pattern(string=w603, regular expression="\r\n") -> (before substring=w600:string, after substring=w602:string, offset past match=w601:i32)  [unwired: 1 in, 1 out]
                    n172 = call <vilib>:"Trim Whitespace.vi"("string"=w600) -> ("trimmed string"=w597:string)  [unwired: 1 in]
                    n173 = Equal?(x=w601, y=-1) -> (x = y?=w604:bool)
                    n174 = To Upper Case(1:w597) -> (0:w595:string)
                    n175 = String Length(string=w595) -> (length=w594:i32)
                    n176 = Greater?(x=w594, y=3) -> (0:w592:bool)
                    n177 = case shown="True" w592 {
                      tunnel: w599 -> [w606 w609]
                      tunnel: [w606 w608] -> w598
                      tunnel: w595 -> [_ w607]
                      frame False {
                      }
                      frame True {
                        n178 = Build Array (concatenate)(w609, w607) -> (w608:string[])
                      }
                    }
                  }
                  n179 = property on="VISA resource name" class="VISAName"(error in=w563) -> (error out=w556:errorcluster, "Value"=w564:refnum<visa-resource-name>)  [unwired: 1 in, 1 out]
                  n180 = Build Array (concatenate)(w549, string[] ["MT", "VR", "SN"] ("array")) -> (w560:string[])
                  n181 = Array Size(array=w560) -> (size(s)=w550:i32)
                  n182 = Bundle By Name(cluster=T12 {"Minimum"=0.0, "Maximum"=0.0, "Increment"=0.0} ("Data Entry Limits"), "Minimum"=0.0, "Maximum"=w550) -> (w558:T12)
                  n183 = property on="Horizontal Progress Bar" class="Slide (strict)"(error in=w556, "Data Range"=w558) -> (error out=w555:errorcluster)  [unwired: 1 in, 1 out]
                  n184 = for {
                    tunnel: w560 -> [w572] mode=indexing
                    tunnel: w564 -> [w582]
                    tunnel: w555 -> [w581]
                    tunnel: [w579] -> w551
                    i -> [w583]
                    n185 = Concatenate Strings(w572, "\r\n" ("string")) -> (w570:string)
                    n186 = VISA Write(VISA resource name=w582, write buffer=w570, error in (no error)=w581) -> (VISA resource name out=w577:refnum<visa-resource-name>, error out=w580:errorcluster)  [unwired: 1 out]
                    n187 = flat-sequence {
                      tunnel: w580 -> [w589]
                      tunnel: [w589] -> w578
                      frame #0 {
                        n188 = Wait (ms)(milliseconds to wait=u32 50) -> ()  [unwired: 1 out]
                      }
                    }
                    n189 = disable-structure shown="Disabled" {
                      disable-tunnel: [w587 _] -> w579
                      disable-tunnel: w578 -> [w586 _]
                      disable-tunnel: w577 -> [w585 _]
                      disable-tunnel: [w584 _] -> w573
                      frame Disabled {
                        n190 = VISA Read(VISA resource name=w585, byte count=u32 16, error in (no error)=w586) -> (read buffer=w584:string, error out=w587:errorcluster)  [unwired: 2 out]
                      }
                      frame Enabled {
                      }
                    }
                    n191 = feedback #2("") -> (w575:string)
                    n192 = Concatenate Strings(w575, w570, w573) -> (w576:string)
                    n193 = feedback-in #2(w576) -> ()
                    n194 = property on="read buffer" class="Str"("Value"=w576) -> ()  [unwired: 2 in, 2 out]
                    "Horizontal Progress Bar" <- w583
                  }
                }
              }
            }
            event "Can Send": Value Change {
              (unwired) u8[] [1, 184, 11, 1, 0, 0, 0, 0] ("Data 2")
              w640 = u8 0 items=["STATUS"=128, "EXTENDED"=2, "RTR"=1, "DATA MSG"=0] ("MSGTYPE")
              w645 = u8 1 items=["Standart flag", "Extern flag"] ("Format")
              w644 = u8 0 items=["Data flag", "Remote flag"] ("Type")
              # "Send"
              n195 = event-data() -> ()  [unwired: 1 in, 6 out]
              n196 = In Range and Coerce(upper limit=u16 18001, x="Motor Speed RPM", lower limit=u16 0) -> (coerced(x)=w626:u16, In Range?=w624:bool)
              n197 = Not(x=w624) -> (.not. x?=w625:bool)
              n198 = Select(t=w626, s=w624, f=u16 0) -> (s? t:f=w628:u16)
              n199 = call "Display Message to User"("Enable"=w625) -> ()  [unwired: 9 in, 2 out]
              n200 = property on="Unit Adress" class="DigNum (strict)"() -> ("Value"=w622:u8)  [unwired: 2 in, 2 out]
              n201 = Split Number(x=w628) -> (hi(x)=w632:u8, lo(x)=w633:u8)
              n202 = case shown="95" w622 {
                tunnel: [w662 w667 w678] -> w638
                tunnel: w633 -> [w661 w666 w677]
                tunnel: w632 -> [w660 w665 w676]
                frame 47, Default {
                  w658 = u8 0 ("element")
                  w659 = u8 1 ("element")
                  n203 = Build Array(w659, w661, w660, w659, w658, w658, w658, w658) -> (w662:u8[])
                }
                frame 63 {
                  w663 = u8 0 ("element")
                  w664 = u8 1 ("element")
                  n204 = Build Array(w664, w666, w665, w664, w663, w663, w663, w663) -> (w667:u8[])
                }
                frame 95 {
                  w674 = u8 0 ("element")
                  n205 = Boolean To (0,1)(Boolean="Speed control") -> (0, 1=w672:i16)
                  n206 = Boolean To (0,1)(Boolean="Motor Over Temp") -> (0, 1=w673:i16)
                  n207 = To Unsigned Byte Integer(number=w672) -> (unsigned 8bit integer=w669:u8)
                  n208 = To Unsigned Byte Integer(number=w673) -> (unsigned 8bit integer=w668:u8)
                  n209 = Build Array(u8 1 ("element"), w677, w676, w669, w668, w674, w674, w674) -> (w678:u8[])
                }
              }
              n210 = case shown="95, Default" w622 {
                tunnel: [u32 417357607 u32 417349415 u32 417345319] -> w623
                frame 95, Default {
                }
                frame 63 {
                }
                frame 47 {
                }
              }
              n211 = Array Size(array=w638) -> (size(s)=w643:i32)
              n212 = call "Array Data to Single Num in Hex.vi"("aDATA"=w638) -> ("Numeric"=→"Data Send":u64)  [unwired: 10 in]
              n213 = To Unsigned Byte Integer(number=w643) -> (unsigned 8bit integer=w641:u8)
              n214 = Bundle By Name(cluster=T10 {"ID"=0, "MSGTYPE"=0, "LEN"=0, "aDATA"=[]} ("MsgTX 2"), "ID"=w623, "MSGTYPE"=w640, "LEN"=w641, "aDATA"=w638) -> (w639:T10)
              n215 = call "CANAnalData.vi"("ID"=w623, "Data"=w638, "Config"=w636) -> ()  [unwired: 4 in, 5 out]
              n216 = Unbundle By Name(w639) -> ("ID"=w653:u32, "LEN"=w654:u8, "aDATA"=w655:u8[])  [unwired: 1 out]
              n217 = property class="Clust (strict)"(reference=w636) -> ("Value"=w652:T8)  [unwired: 1 in, 2 out]
              n218 = Bundle By Name(cluster=T13 {"ID"=0, "TimeStamp"=0, "TimeFlag"=0, "SendType"=0, "RemoteFlag"=0, "ExternFlag"=0, "DataLen"=0, "Data"=[], "Reserved"=[]} ("Send"), "ID"=w653, "RemoteFlag"=w644, "ExternFlag"=w645, "DataLen"=w654, "Data"=w655) -> (w650:T13)
              n219 = Unbundle By Name(w652) -> ("DevType"=w646:T2, "DevIndex"=w647:u32, "CanIndex"=w648:T3)
              n220 = Build Array(w650) -> (w649:T13[])
              n221 = call "VCI_Transmit.vi"("Buffer"=w649, "CANIndex"=w648, "DevIndex"=w647, "DevType"=w646) -> ()  [unwired: 1 in, 7 out]
            }
            event "Graph Button": Value Change {
              n222 = event-data() -> ()  [unwired: 1 in, 6 out]
              n223 = Not(x="Graph Button") -> (.not. x?=w683:bool)
              n224 = property on="Array" class="Arr (strict)"("Visible"=w683) -> (error out=w682:errorcluster)  [unwired: 2 in, 1 out]
              n225 = property on="Waveform Chart" class="WFChart (strict)"(error in=w682, "Visible"="Graph Button") -> ()  [unwired: 1 in, 2 out]
            }
            event "Serial Com": Value Change {
              n226 = event-data() -> ()  [unwired: 1 in, 6 out]
              n227 = property on="Serial Com" class="Bool"(error in=w693, "Visible"=FALSE) -> (error out=w692:errorcluster)  [unwired: 1 in, 1 out]
              n228 = property on="VISA resource name" class="VISAName"(error in=w692, "Visible"=TRUE) -> (error out=w690:errorcluster)  [unwired: 1 in, 1 out]
            }
            event "VISA resource name": Value Change {
              n229 = event-data() -> ()  [unwired: 1 in, 1 out]
              n230 = call "Serial Init.vi"("error in (no error)"=w704, "VISA Refnum in"="VISA resource name") -> ("error out"=w713:errorcluster, "Boolean"=w700:bool)  [unwired: 8 in]
              n231 = property on="Serial Status" class="Bool (strict)"(error in=w713, "Value"=w700) -> (error out=w707:errorcluster)  [unwired: 1 in, 1 out]
              n232 = property on="VISA resource name" class="VISAName"(error in=w707, "Visible"=FALSE) -> (error out=w706:errorcluster)  [unwired: 1 in, 1 out]
              n233 = property on="Serial Com" class="Bool"(error in=w706, "Visible"=TRUE) -> (error out=w703:errorcluster)  [unwired: 1 in, 1 out]
              n234 = call <vilib>:"Clear Errors.vi"("error in (no error)"=w703) -> ("error out"=w702:errorcluster)  [unwired: 5 in, 1 out]
              n235 = case shown="True" w700 {
                tunnel: w702 -> [w714 w717]
                tunnel: [w714 w716] -> w701
                tunnel: "VISA resource name" -> [_ w715]
                frame False {
                }
                frame True {
                  n236 = VISA Flush I/O Buffer(VISA resource name=w715, error in (no error)=w717) -> (error out=w716:errorcluster)  [unwired: 1 in, 1 out]
                }
              }
            }
            event "Stop": Value Change {
              n237 = event-data() -> ()  [unwired: 1 in, 6 out]
              n238 = Flush Queue(queue=w722, error in (no error)=w721) -> (queue out=w720:refnum<queue>, error out=w719:errorcluster)  [unwired: 1 out]
              n239 = Release Queue(queue=w720, error in (no error)=w719) -> (error out=w718:errorcluster)  [unwired: 1 in, 2 out]
            }
            event "Refresh Button": Value Change {
              n240 = event-data() -> ()  [unwired: 1 in, 6 out]
              n241 = Release Queue(queue=w727, error in (no error)=w728) -> (error out=w726:errorcluster)  [unwired: 1 in, 2 out]
            }
          }
          n242 = Unbundle By Name(w210) -> ("status"=w216:bool)
          n243 = Or(x=w216, y=w208) -> (x .or. y?=w215:bool)
        }
        n244 = while {
          shift-right: [w95] -> _
          shift-left: w81 -> [w97]
          shift-right: [w93] -> _
          shift-left: _ -> [w94]
          shift-right: [w90] -> _
          shift-left: dbl[] [] -> [w89]
          shift-right: [w87] -> _
          shift-left: w80 -> [w87]
          stop <- w96 stop-if-true
          # "Consumer Loop"
          n245 = Dequeue Element(queue=w97, error in (no error)=w87) -> (queue out=w95:refnum<queue>, element=w88:T9, error out=w96:errorcluster)  [unwired: 1 in, 1 out]
          n246 = for {
            tunnel: [w203] -> w92 mode=indexing
            tunnel: w88 -> [w202] mode=indexing
            tunnel: [w201] -> w91 mode=indexing
            n247 = Unbundle By Name(w202) -> ("aDATA"=w201:u8[])
            n248 = call "Array Data to Single Num in Hex.vi"("aDATA"=w201) -> ("Numeric"=w203:u64)  [unwired: 10 in]
          }
          n249 = Build Array (concatenate)(w92, w94) -> (w93:u64[][])
          "Array" <- w93
          n250 = for {
            tunnel: w91 -> [w102] mode=indexing
            tunnel: [w100] -> w90
            tunnel: w89 -> [w99]
            tunnel: w88 -> [w98]
            i -> [w101]
            n251 = case shown="1" w101 {
              tunnel: w102 -> [w136 w169 w200]
              tunnel: [w110 w164 w194] -> w100
              tunnel: w99 -> [w111 w164 w194]
              tunnel: w98 -> [w109 _ _]
              frame 0, Default {
                # "Frame ID\n0x18E1273F"
                n252 = Index Array(array=w136, index #1=0 ("index"), index #2=1 ("index"), index #3=2 ("index"), index #4=3 ("index"), index #5=4 ("index"), index #6=5 ("index"), index #7=6 ("index"), index #8=7 ("index")) -> (element #1=w120:u8, element #2=w122:u8, element #3=w123:u8, element #4=w127:u8, element #5=w130:u8, element #6=w134:u8, element #7=w135:u8, element #8=w133:u8)
                n253 = Join Numbers(hi=w135, lo=w134) -> ((hi.lo)=w154:u16)
                n254 = Join Numbers(hi=w123, lo=w122) -> ((hi.lo)=w124:u16)
                n255 = Number To Hexadecimal String(2:w130) -> (0:w131:string)  [unwired: 1 in]
                n256 = Number To Hexadecimal String(2:w154) -> (0:w153:string)  [unwired: 1 in]
                n257 = Number To Hexadecimal String(2:w120) -> (0:w121:string)  [unwired: 1 in]
                n258 = Number To Hexadecimal String(2:w124) -> (0:w125:string)  [unwired: 1 in]
                n259 = Number To Hexadecimal String(2:w127) -> (0:w128:string)  [unwired: 1 in]
                n260 = Number To Hexadecimal String(2:w133) -> (0:w147:string)  [unwired: 1 in]
                n261 = Hexadecimal String To Number(string=w131) -> (number=w132:u32)  [unwired: 2 in, 1 out]
                n262 = Hexadecimal String To Number(string=w153) -> (number=w152:u32)  [unwired: 2 in, 1 out]
                n263 = Hexadecimal String To Number(string=w121) -> (number=w118:u32)  [unwired: 2 in, 1 out]
                n264 = Hexadecimal String To Number(string=w125) -> (number=w126:u32)  [unwired: 2 in, 1 out]
                n265 = Hexadecimal String To Number(string=w128) -> (number=w129:u32)  [unwired: 2 in, 1 out]
                n266 = Hexadecimal String To Number(string=w147) -> (number=w146:u32)  [unwired: 2 in, 1 out]
                n267 = To Double Precision Float(number=u32 10 ("y")) -> (double precision float=w150:dbl)
                n268 = To Double Precision Float(number=w152) -> (double precision float=w149:dbl)
                n269 = To Double Precision Float(number=w132) -> (double precision float=w113:dbl)
                n270 = To Double Precision Float(number=w126) -> (double precision float=w106:dbl)
                "Motor Speed RPM" <- w106
                n271 = To Double Precision Float(number=w129) -> (double precision float=w115:dbl)
                n272 = To Double Precision Float(number=w146) -> (double precision float=→"DC Current":dbl)
                n273 = Divide(x=w149, y=w150) -> (x/y=→"DC Voltage":dbl)
                n274 = To Unsigned Word Integer(number=w118) -> (unsigned 16bit integer=→"ECS State":u16)
                n275 = Subtract(x=w113, y=50.0 ("x")) -> (x-y=→"Power transistor Heat sink Temp.":dbl)
                n276 = Subtract(x=w115, y=50.0 ("x")) -> (x-y=→"Motor Stator Temp.":dbl)
                n277 = Index Array(array=w109, index=0) -> (element=w107:T10)
                n278 = Unbundle By Name(w107) -> ("ID"=w105:u32)
                n279 = Equal?(x=u32 417408815, y=w105) -> (x = y?=w103:bool)
                n280 = case shown="True" w103 {
                  tunnel: w111 -> [w155 w158]
                  tunnel: [w155 w157] -> w110
                  tunnel: w106 -> [_ w156]
                  frame False {
                  }
                  frame True {
                    n281 = call "Write To Measurement File2"("Signals"=w156) -> ()  [unwired: 16 in, 3 out]
                    n282 = Build Array (concatenate)(w156, w158) -> (w157:dbl[])
                    "Waveform Chart" <- w157
                  }
                }
              }
              frame 1 {
                # "Framde ID\n0x18E3273F"
                n283 = Index Array(array=w169, index #1=0 ("index"), index #2=1 ("index")) -> (element #1=w167:u8, element #2=w161:u8)
                n284 = Number To Boolean Array(number=w167) -> (Boolean array=w166:bool[])
                n285 = Number To Boolean Array(number=w161) -> (Boolean array=w163:bool[])
                n286 = Boolean To (0,1)(Boolean=w166) -> (0, 1=w165:i16[])
                n287 = Boolean To (0,1)(Boolean=w163) -> (0, 1=w160:i16[])
                n288 = for {
                  tunnel: w165 -> [w179] mode=indexing
                  i -> [w180]
                  n289 = Not Equal To 0?(x=w179) -> (x != 0?=w178:bool)
                  n290 = case shown="0, Default" w180 {
                    tunnel: w178 -> [w181 w182 w183 w184 w185 w186 w187 w188]
                    frame 0, Default {
                      "Drive Sensor temp Failure" <- w181
                    }
                    frame 1 {
                      "Drive Over temperature" <- w182
                    }
                    frame 2 {
                      "Motor Sensor temp Fauilre" <- w183
                    }
                    frame 3 {
                      "Motor Over temperature" <- w184
                    }
                    frame 4 {
                      "Derated drive temp" <- w185
                    }
                    frame 5 {
                      "Under voltage/Over voltage" <- w186
                    }
                    frame 6 {
                      "Commutation err" <- w187
                    }
                    frame 7 {
                      "Speed error" <- w188
                    }
                  }
                }
                n291 = property on="Unit Adress" class="DigNum (strict)"() -> ("Value"=w159:u8)  [unwired: 2 in, 2 out]
                n292 = case shown="95" w159 {
                  tunnel: w160 -> [_ w170]
                  frame 0, Default {
                  }
                  frame 95 {
                    n293 = for {
                      tunnel: w170 -> [w175] mode=indexing
                      i -> [w171]
                      stop <- w173 stop-if-true
                      n294 = Not Equal To 0?(x=w175) -> (x != 0?=w174:bool)
                      n295 = case shown="0, Default" w171 {
                        tunnel: w174 -> [w176 w177]
                        frame 0, Default {
                          "Ambient Sensor temp" <- w176
                        }
                        frame 1 {
                          "Ambient Over temp" <- w177
                        }
                      }
                      n296 = Equal?(x=w171, y=1.0) -> (x = y?=w173:bool)
                    }
                  }
                }
              }
              frame 2 {
                # "Frame ID\n0x18E2273F"
                n297 = Index Array(array=w200, index #1=0 ("index"), index #2=1 ("index")) -> (element #1=w197:u8, element #2=w192:u8)
                n298 = Number To Hexadecimal String(2:w197) -> (0:w196:string)  [unwired: 1 in]
                n299 = Number To Hexadecimal String(2:w192) -> (0:w190:string)  [unwired: 1 in]
                n300 = Hexadecimal String To Number(string=w190) -> (number=w191:u32)  [unwired: 2 in, 1 out]
                n301 = Hexadecimal String To Number(string=w196) -> (number=w198:u32)  [unwired: 2 in, 1 out]
                n302 = To Double Precision Float(number=w191) -> (double precision float=→"Ambient Temperature":dbl)
                n303 = To Double Precision Float(number=w198) -> (double precision float=→"Motor Phase Current RMS":dbl)
              }
            }
          }
        }
      }
      frame "Stop" {
        n304 = Release Queue(queue=w735, error in (no error)=w737) -> (error out=w736:errorcluster)  [unwired: 1 in, 2 out]
        n305 = flat-sequence {
          tunnel: w734 -> [w746]
          tunnel: [TRUE ("Stop")] -> w733
          frame #0 {
            w745 = u8[] [1, 0, 0, 0, 0, 0, 0, 0] ("Data 2")
            w748 = u8 0 items=["STATUS"=128, "EXTENDED"=2, "RTR"=1, "DATA MSG"=0] ("MSGTYPE")
            w753 = u8 1 items=["Standart flag", "Extern flag"] ("Format")
            w752 = u8 0 items=["Data flag", "Remote flag"] ("Type")
            n306 = property on="Serial Status" class="Bool (strict)"() -> ("Value"=w738:bool)  [unwired: 2 in, 2 out]
            n307 = property on="Unit Adress" class="DigNum (strict)"() -> ("Value"=w740:u8)  [unwired: 2 in, 2 out]
            n308 = case shown="True" w738 {
              frame False {
              }
              frame True {
                n309 = property on="VISA resource name" class="VISAName"() -> ("Value"=w764:refnum<visa-resource-name>)  [unwired: 2 in, 2 out]
                n310 = VISA Close(VISA resource name=w764) -> ()  [unwired: 1 in, 1 out]
              }
            }
            n311 = case shown="95, Default" w740 {
              tunnel: [u32 417357607 u32 417349415 u32 417345319] -> w739
              frame 95, Default {
              }
              frame 63 {
              }
              frame 47 {
              }
            }
            n312 = property on="Graph Button" class="Bool (strict)"("Value"=FALSE ("Graph Button")) -> ()  [unwired: 2 in, 2 out]
            n313 = Array Size(array=w745) -> (size(s)=w751:i32)
            n314 = To Unsigned Byte Integer(number=w751) -> (unsigned 8bit integer=w749:u8)
            n315 = property on="Waveform Chart" class="WFChart (strict)"("Visible"=FALSE, "Value"=dbl[] [] ("Waveform Chart")) -> ()  [unwired: 2 in, 2 out]
            n316 = Bundle By Name(cluster=T10 {"ID"=0, "MSGTYPE"=0, "LEN"=0, "aDATA"=[]} ("MsgTX 2"), "ID"=w739, "MSGTYPE"=w748, "LEN"=w749, "aDATA"=w745) -> (w747:T10)
            n317 = call "CANAnalData.vi"("ID"=w739, "Data"=w745, "Config"=w746) -> ()  [unwired: 4 in, 5 out]
            n318 = call "Array Data to Single Num in Hex.vi"("aDATA"=w745) -> ("Numeric"=w744:u64)  [unwired: 10 in]
            n319 = property on="Data Send" class="DigNum (strict)"("Value"=w744) -> ()  [unwired: 2 in, 2 out]
            n320 = Unbundle By Name(w747) -> ("ID"=w761:u32, "LEN"=w762:u8, "aDATA"=w763:u8[])  [unwired: 1 out]
            n321 = property class="Clust (strict)"(reference=w746) -> ("Value"=w760:T8)  [unwired: 1 in, 2 out]
            n322 = Bundle By Name(cluster=T13 {"ID"=0, "TimeStamp"=0, "TimeFlag"=0, "SendType"=0, "RemoteFlag"=0, "ExternFlag"=0, "DataLen"=0, "Data"=[], "Reserved"=[]} ("Send"), "ID"=w761, "RemoteFlag"=w752, "ExternFlag"=w753, "DataLen"=w762, "Data"=w763) -> (w758:T13)
            n323 = Unbundle By Name(w760) -> ("DevType"=w754:T2, "DevIndex"=w755:u32, "CanIndex"=w756:T3)
            n324 = Build Array(w758) -> (w757:T13[])
            n325 = call "VCI_Transmit.vi"("Buffer"=w757, "CANIndex"=w756, "DevIndex"=w755, "DevType"=w754) -> ()  [unwired: 1 in, 7 out]
          }
          frame #1 {
          }
        }
      }
    }
  }
  n326 = disable-structure shown="Disabled" {
    frame Disabled {
      n327 = property on="Serial Send" class="Bool" props=["Visible"]() -> ()  [unwired: 2 in, 3 out]
      n328 = property on="Speed control" class="Bool (strict)" props=["Visible"]() -> ()  [unwired: 3 in, 2 out]
      n329 = property on="Motor Over Temp" class="Bool (strict)" props=["Visible"]() -> ()  [unwired: 3 in, 2 out]
      n330 = property on="Set Param." class="Bool" props=["Visible"]() -> ()  [unwired: 2 in, 3 out]
      n331 = property on="Unit Adress" class="DigNum (strict)" props=["Visible"]() -> ()  [unwired: 3 in, 2 out]
      n332 = property on="Set Param." class="Bool" props=["Visible"]() -> ()  [unwired: 3 in, 2 out]
      n333 = property on="Msg Count" class="DigNum (strict)" props=["Visible"]() -> ()  [unwired: 3 in, 2 out]
      n334 = property on="Param to Set" class="Ring (strict)" props=["Visible"]() -> ()  [unwired: 3 in, 2 out]
      n335 = property on="Ambient Temperature" class="DigNum (strict)" props=["Visible"]() -> ()  [unwired: 3 in, 2 out]
      n336 = property on="Ambient Over temp" class="Bool (strict)" props=["Visible"]() -> ()  [unwired: 3 in, 2 out]
      n337 = property on="Ambient Sensor temp" class="Bool (strict)" props=["Visible"]() -> ()  [unwired: 3 in, 2 out]
    }
    frame Enabled {
    }
  }
